vi "listen_tcp_data_conn.vi"(8 "error in":errorcluster, 9 "TCP output port":i32=6666, 10 "TCP input port":i32=6666) -> (0 "error out":errorcluster)   [LabVIEW 2014]
uses:
  main/ilemt_globals.vi
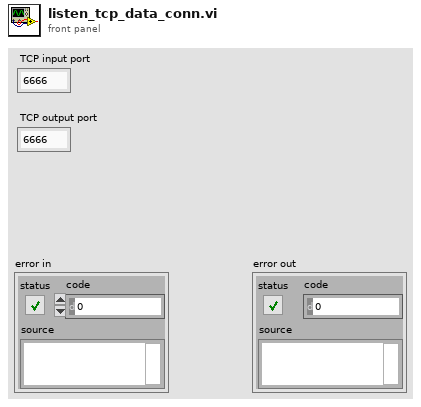
[diagram p1: front panel]
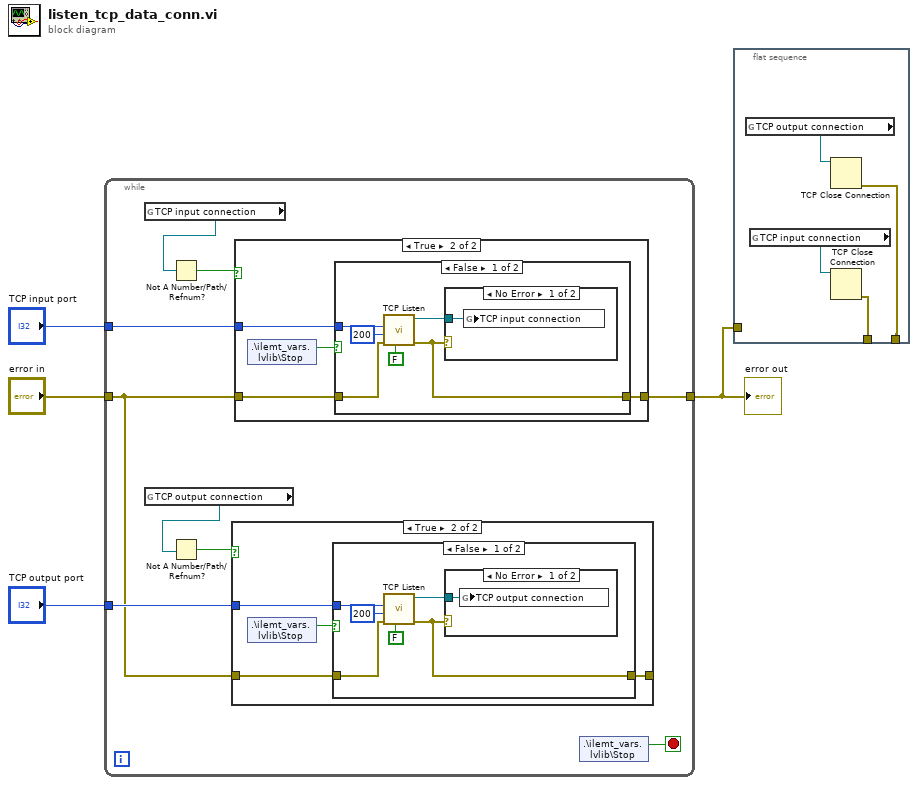
[diagram p0: block diagram]
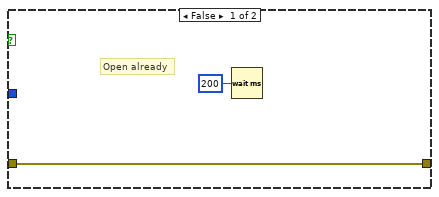
[diagram p2: hidden frame]
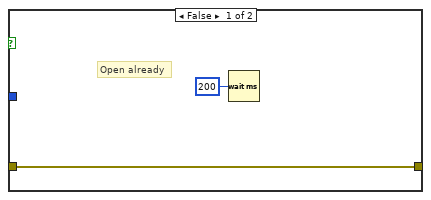
[diagram p5: hidden frame]
diagram:
  n1 = while {
    tunnel: "TCP input port" -> [w11]
    tunnel: "error in" -> [w6]
    tunnel: [w10] -> w2
    tunnel: "TCP output port" -> [w7]
    stop <- w9 stop-if-true
    n2 = global read "ilemt_globals.vi" "TCP input connection"() -> (w13:refnum<k5>)
    n3 = global read "ilemt_globals.vi" "TCP output connection"() -> (w5:refnum<k5>)
    n4 = Not A Number/Path/Refnum?(number/path/refnum=w13) -> (NaN/Path/Refnum?=w12:bool)
    n5 = Not A Number/Path/Refnum?(number/path/refnum=w5) -> (NaN/Path/Refnum?=w8:bool)
    n6 = case shown="True" w8 {
      tunnel: w7 -> [_ w19]
      tunnel: w6 -> [w15 w18]
      tunnel: [w15 w17] -> _
      frame False {
        # "Open already"
        n7 = Wait (ms)(milliseconds to wait=u32 200) -> ()  [unwired: 1 out]
      }
      frame True {
        n8 = shared-variable ".\\ilemt_vars.lvlib\\Stop"() -> (w16:bool)  [unwired: 1 in, 1 out]
        n9 = case shown="False" w16 {
          tunnel: w19 -> [w25 _]
          tunnel: w18 -> [w23 w27]
          tunnel: [w20 w27] -> w17
          frame False {
            n10 = call <vilib>:"TCP Listen.vi"("resolve remote address (T)"=FALSE, "error in (no error)"=w23, "timeout ms (wait forever: -1)"=200, "port"=w25) -> ("error out"=w20:errorcluster, "connection ID"=w21:refnum<k5>)  [unwired: 3 in, 3 out]
            n11 = case shown="No Error" w20 {
              tunnel: w21 -> [w26 _]
              frame No Error {
                n12 = global write "ilemt_globals.vi" "TCP output connection"(w26) -> ()
              }
              frame Error {
              }
            }
          }
          frame True {
          }
        }
      }
    }
    n13 = case shown="True" w12 {
      tunnel: w11 -> [_ w33]
      tunnel: w6 -> [w29 w32]
      tunnel: [w29 w31] -> w10
      frame False {
        # "Open already"
        n14 = Wait (ms)(milliseconds to wait=u32 200) -> ()  [unwired: 1 out]
      }
      frame True {
        n15 = shared-variable ".\\ilemt_vars.lvlib\\Stop"() -> (w30:bool)  [unwired: 1 in, 1 out]
        n16 = case shown="False" w30 {
          tunnel: w33 -> [w39 _]
          tunnel: w32 -> [w37 w41]
          tunnel: [w34 w41] -> w31
          frame False {
            n17 = call <vilib>:"TCP Listen.vi"("resolve remote address (T)"=FALSE, "error in (no error)"=w37, "timeout ms (wait forever: -1)"=200, "port"=w39) -> ("error out"=w34:errorcluster, "connection ID"=w35:refnum<k5>)  [unwired: 3 in, 3 out]
            n18 = case shown="No Error" w34 {
              tunnel: w35 -> [w40 _]
              frame No Error {
                n19 = global write "ilemt_globals.vi" "TCP input connection"(w40) -> ()
              }
              frame Error {
              }
            }
          }
          frame True {
          }
        }
      }
    }
    n20 = shared-variable ".\\ilemt_vars.lvlib\\Stop"() -> (w9:bool)  [unwired: 1 in, 1 out]
  }
  "error out" <- w2
  n21 = flat-sequence {
    tunnel: w2 -> [_]
    tunnel: [w44] -> _
    tunnel: [w42] -> _
    frame #0 {
      n22 = global read "ilemt_globals.vi" "TCP output connection"() -> (w43:refnum<k5>)
      n23 = global read "ilemt_globals.vi" "TCP input connection"() -> (w45:refnum<k5>)
      n24 = TCP Close Connection(connection ID=w43) -> (error out=w42:errorcluster)  [unwired: 1 in, 2 out]
      n25 = TCP Close Connection(connection ID=w45) -> (error out=w44:errorcluster)  [unwired: 1 in, 2 out]
    }
  }
